vi "dataAcq_get_interferogram_part.vi"(0 "reference":refnum<class "OSA.lvclass">, 5 "error in (no error)":errorcluster) -> (14 "duplicate reference":refnum<class "OSA.lvclass">, 19 "error out":errorcluster)   [LabVIEW 2010, in "OSA.lvclass"]
doc: "Reads data from spectrometer and updates interferogram Y array, X is equidistant and only x min and max are retrieved. \n\nX: optical path length\nY: ADC value\n\nServes mainly compatibility issues - not recommended for new design/vis."
uses:
  OSA.lvclass
  OSA20X_misc.lvlib
  FTSLib.dll
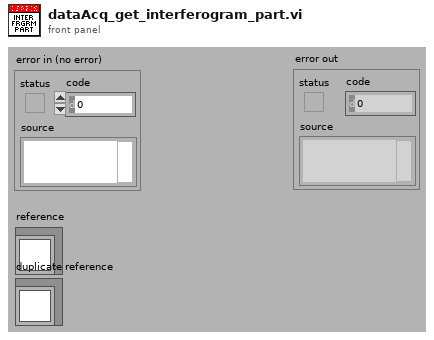
[diagram p1: front panel]
types:
  T1 = enum16{"get", "init", "set interferogram", "set spectrum", "cleanUp"}
  T2 = typedef "OSA.lvclass/ObjectAttributes.ctl" = cluster{"Stop":bool, "dataType":T3, "spectrometerIdx":u16, "buffer size interferogram":i32, "interferogram":cluster{"new":bool, "plot_x_ min":sgl, "plot_x_max":sgl, "plot_y_min":sgl, "plot_y_max":sgl, "Graph Intrfrgrm":T4, "timeStamp":u32, "signal (%)":dbl, "traces":cluster{"idx":u32, "broadBand":bool, "monoChromatic":bool, "peakToPeakSignal":dbl, "peakToPeakPos":dbl}[], "traces idx last":i32}, "spectrum":cluster{"new":bool, "plot_x_min":sgl, "plot_x_max":sgl, "plot_unit_x":T5, "plot_unit_y":T6, "plot_y_min":sgl, "plot_y_max":sgl, "Graph Spectrum":T4, "timeStamp":u32, "X_VAL_OPTIONS":enum16{"MIN_MAX", "ARRAY"}, "traces":cluster{"idx":u32}[], "traces idx last":i32}, "Thorlabs_OSA_64.lvclass:queue_action.ctlqueue ref":refnum<queue>, "action":T7, "plot zoom step":dbl, "buffer semaphore":T8, "acq stopped":bool, "dataType active":T3, "temperature (degr C)":sgl, "pressure (hPa)":sgl, "rel humidity (%)":sgl, "settings":cluster{"resolution":u16, "sensitivity":u16, "Average":bool, "average nr":u32, "apodisation":T9, "acq delay (ms)":u32, "airMesure":T10, "wmtr on":bool, "intfgrm_smooth_width":u16, "intfgrm_smooth_nrOfPasses":u16, "intfgrm_smooth":T11, "phaseCorrection":T12, "zeroFill":u8, "spectr_smooth":T11, "spectr_smooth_width":u16, "spectr_smooth_nrOfPasses":u16, "resolution (/cm)":sgl, "REF wavelength, (nm)":dbl, "gain_idx":u16, "gainAuto":bool, "gain_relative":dbl, "PD sensitivity mode":T13, "PD senseMode implemented":bool, "SensorTemperature implemented":bool, "SensorPressure implemented":bool, "SensorHumidity implemented":bool}, "peaks position":sgl[], "peaks width":sgl[], "peaks height":sgl[], "peaks max nr":u32, "peaks latest nr":i32, "peaks new":bool, "power":dbl, "power new":bool, "path":string, "wavelength (WNr)":dbl, "wavelength new":bool, "buffer size spectrum":i32, "status":string, "VI reference":refnum<vi>, "funcPointer":u64, "libraryPointer":u64, "singleAcquisition":bool, "coherenceLength (cm)":dbl, "coherenceLength new":bool, "spectrometer model":string, "spectrometer serial nr":string, "peaks thld left":sgl[], "peaks thld right":sgl[], "coherenceLength error (cm)":dbl, "ADC bits":u16, "peaks position centroid":sgl[], "peaks height centroid":sgl[], "OSA series":T14, "channel index spectrum":u16, "spectrometer rangeLow, (/cm)":dbl, "spectrometer rangeHigh, (/cm)":dbl, "channel index interferogram":u16}
  T3 = typedef "OSA.lvclass/acq_dataType.ctl" = enum16{"none", "interferogram", "spectrum"}
  T4 = typedef "OSA.lvclass/graph_intensity.ctl" = refnum<vi>
  T5 = typedef "OSA.lvclass/spectrum_x_unit.ctl" = enum16{"wavenr/cm", "THz", "eV", "nm_air", "nm_vac"}
  T6 = typedef "OSA.lvclass/y_unit.ctl" = enum16{"ADC counts", "dBm pwr absolute", "dBm pwr density", "mW pwr absolute", "mW pwr density"}
  T7 = typedef "OSA.lvclass/queue_action.ctl" = enum16{"none", "stop", "GUI_plotInterferogram", "GUI_plotSpectrum", "GUI_plotInterferogramRescale", "GUI_plotSpectrumRescale", "GUI_plotInterferogramReset", "GUI_plotSpectrumReset", "GUI_plotInterferogramAutoScaleY", "GUI_plotSpectrumAutoScaleY", "GUI_plotInterferogramZoomOut", "GUI_plotSpectrumZoomOut", "GUI_plotInterferogramPane", "GUI_plotSpectrumPane", "GUI_plotInterferogramZoomMouse", "GUI_plotSpectrumZoomMouse", "ENVIRONMENT temperature", "ENVIRONMENT pressure", "MODE_resolution set", "MODE_resolution get", "MODE_sensitivity set", "MODE_sensitivity get", "MODE_PDTemperature set", "MODE_PDTemperature get", "REBOOT/RESET firmware", "ACQASYNC_acquireSingleSpectrum", "ACQASYNC_continuous start", "ACQASYNC_continuous stop\n", "ACQASYNC_get last interferogram", "ACQASYNC_get last spectrum", "ACQASYNC_get last waveNr", "ACQOPT_interferogram smoothing set", "ACQOPT_interferogram smoothing get", "ACQOPT_spectrum smoothing set", "ACQOPT_spectrum smoothing get", "ACQOPT_apodisation type set", "ACQOPT_apodisation type get", "ACQOPT_phase correction type set", "ACQOPT_phase correction type get", "ACQOPT_acqIntervall_set", "ACQOPT_acqIntervall_get", "ACQOPT_average spectrum set", "ACQOPT_average spectrum get", "ACQOPT_rolling average set", "ACQOPT_rolling average get", "ACQOPT_zero fill factor set", "ACQOPT_zero fill factor get", "ACQOPT_cycle counting set", "ACQOPT_cycle counting get", "ACQOPT_air measure option set", "ACQOPT_air measure option get", "ACQOPT_gainLevel auto get", "ACQOPT_gainLevel auto set", "ACQOPT_gainLevel get", "ACQOPT_gainLevel set", "ACQOPT_getAll", "INSTRUMENT_PROPERTY_range_WaveNr_min", "INSTRUMENT_PROPERTY_range_WaveNr_max", "INSTRUMENT_PROPERTY_reference_wavelength_cm^-1", "INSTRUMENT_PROPERTY_samplesPerRefPeriod", "INSTRUMENT_PROPERTY_resolution_waveNrPercm", "INSTRUMENT_PROPERTY_availableGainLevels", "INSTRUMENT_PROPERTY_status", "CONVERT", "ANALYSE_POWER", "ANALYSE_PEAKS", "ANALYSE_WAVELENGTH", "ANALYSE_SPECTRUM", "ANALYSE_INTERFEROGRAM", "ANALYSE_COHERENCE_LENGTH", "MATH", "MATH_power", "MATH_peaks", "FILE", "miscellaneous"}
  T8 = typedef "Semaphore RefNum" = refnum<k1>
  T9 = typedef "OSA.lvclass/apodisation.ctl" = enum16{"NONE", "NORTON_BEER_WEAK", "NORTON_BEER_MEDIUM", "NORTON_BEER_STRONG", "TRIANGULAR", "COSINE", "HANN", "HAMMING", "BLACKMANHARRIS3", "BLACKMANHARRIS4", "GAUSSIAN"}
  T10 = typedef "OSA.lvclass/airMeasure.ctl" = enum16{"TEMPERATURE", "PRESSURE"}
  T11 = typedef "OSA20X_misc.lvlib/interferogram_smoothing.ctl" = enum16{"NONE", "BINOMIAL", "SAVITSKY_GOLAY", "FOURIER", "MOVING_AVERAGE", "GAUSSIAN"}
  T12 = typedef "OSA.lvclass/phaseCorrection.ctl" = enum16{"NONE", "MERTZ", "FORMAN", "MERTZ_FILE", "FORMAN_FILE", "FUTURE COMP."}
  T13 = typedef "OSA20X_misc.lvlib/PDTemperatureMode.ctl" = enum16{"cool: better sensitivity/noise floor", "warm: extended wl range"}
  T14 = typedef "OSA.lvclass/OSA_series.ctl" = enum16{"OSA200", "OSA300", "UNKNOWN"}
  T15 = cluster{"length":u32, "X min (cm)":sgl, "X max (cm)":sgl, "saturated":bool, "broadband":bool, "isMonoChromatic":bool, "peakToPeak, (counts)":dbl, "peakToPeak position (cm)":dbl, "samplesPerRefPeriod":i32}
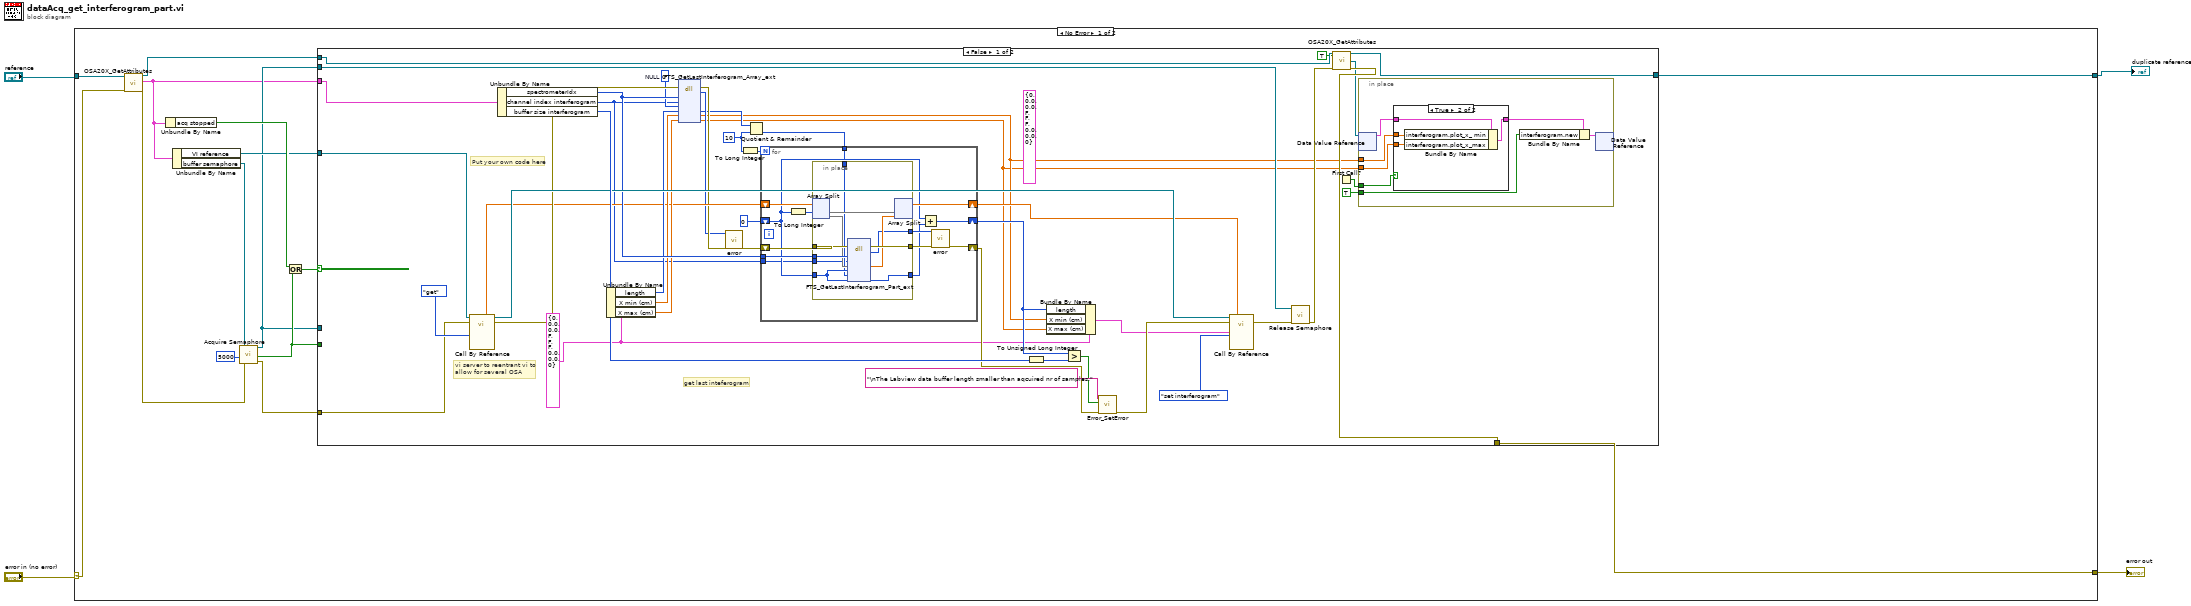
[diagram p0: block diagram]
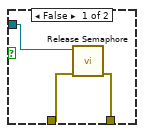
[diagram p4: hidden frame]
diagram:
  n1 = case shown="No Error" "error in (no error)" {
    selector: "error in (no error)" -> [w18 w110]
    tunnel: [w17 w110] -> w3
    tunnel: "reference" -> [w19 w109]
    tunnel: [w16 w109] -> w1
    frame No Error {
      n2 = call "OSA20X_GetAttributes.vi"("reference in"=w19, "error in (no error)"=w18) -> ("reference out"=w8:refnum<class "OSA.lvclass">, "Data"=w5:T2, "error out"=w12:errorcluster)  [unwired: 14 in, 1 out]
      n3 = Unbundle By Name(w5) -> ("acq stopped"=w15:bool)
      n4 = Unbundle By Name(w5) -> ("VI reference"=w9:refnum<vi>, "buffer semaphore"=w13:T8)
      n5 = call <vilib>:"Acquire Semaphore.vi"("error in (no error)"=w12, "ms timeout (-1)"=5000, "semaphore"=w13) -> ("error out"=w10:errorcluster, "timed out"=w7:bool, "semaphore out"=w6:T8)  [unwired: 2 in]
      n6 = Or(x=w15, y=w7) -> (x .or. y?=w14:bool)
      n7 = case shown="False" w14 {
        tunnel: w5 -> [w63 _]
        tunnel: w10 -> [w50 w101]
        tunnel: [w60 w100] -> w17
        tunnel: [w59 w104] -> w16
        tunnel: w6 -> [w52 _]
        tunnel: w9 -> [w49 _]
        tunnel: w8 -> [w47 w104]
        tunnel: w7 -> [_ w103]
        tunnel: w6 -> [_ w102]
        frame False {
          w22 = T15 {"length"=0, "X min (cm)"=0.0, "X max (cm)"=0.0, "saturated"=FALSE, "broadband"=FALSE, "isMonoChromatic"=FALSE, "peakToPeak, (counts)"=0.0, "peakToPeak position (cm)"=0.0, "samplesPerRefPeriod"=0} ("interferogram prop set")
          (unwired) T15 {"length"=0, "X min (cm)"=0.0, "X max (cm)"=0.0, "saturated"=FALSE, "broadband"=FALSE, "isMonoChromatic"=FALSE, "peakToPeak, (counts)"=0.0, "peakToPeak position (cm)"=0.0, "samplesPerRefPeriod"=0} ("interferogram prop set")
          w34 = u32 10 ("y")
          w40 = i64 0  # NULL
          # "get last inteferogram"
          # "vi server to reentrant vi to \nallow for several OSA"
          # "Put your own code here"
          n8 = call-by-ref "?"(reference=w49, error in=w50, "action"=T1."get") -> (reference out=w48:refnum<vi>, error out=w41:errorcluster, "interferogram"=w36:sgl[])  [unwired: 14 in, 4 out]
          n9 = Unbundle By Name(w63) -> ("spectrometerIdx"=w42:u16, "channel index interferogram"=w20:u16, "buffer size interferogram"=w58:i32)
          n10 = Unbundle By Name(w22) -> ("length"=w37:u32, "X min (cm)"=w39:sgl, "X max (cm)"=w38:sgl)
          n11 = dll-call lib="FTSLib.dll" fn="FTS_GetLastInterferogram_Array_ext"(error in=w41, "spectrIdx"=w42, "channel"=w20, "spec"=w40, "length"=w37, "x_min"=w39, "x_max"=w38) -> (error out=w32:errorcluster, "return type"=w30:i32, "length"=w27:u32, "x_min"=w24:sgl, "x_max"=w23:sgl)  [unwired: 5 in, 1 out]
          n12 = call "error.vi"("result code"=w30, "error in (no error)"=w32) -> ("error out"=w31:errorcluster)  [unwired: 15 in, 2 out]
          n13 = To Long Integer(number=w34) -> (32bit integer=w28:i32)
          n14 = Quotient & Remainder(x=w27, y=w34) -> (floor(x/y)=w29:u32)  [unwired: 1 out]
          n15 = for {
            N: w28 -> [_]
            tunnel: w42 -> [w73]
            shift-right: [w75] -> w35
            shift-left: w36 -> [w76]
            shift-right: [w71] -> w25
            shift-left: w31 -> [w74]
            shift-right: [w66] -> w26
            shift-left: u32 0 ("y") -> [w67]
            tunnel: w29 -> [w65]
            tunnel: w20 -> [w64]
            n16 = To Long Integer(number=w67) -> (32bit integer=w70:i32)
            n17 = in-place {
              in-place-border: w73 -> [w87]
              in-place-border: w74 -> [w86]
              in-place-border: [w85] -> w72
              in-place-border: [w81] -> w69
              in-place-border: [w80] -> w68
              in-place-border: w67 -> [w79]
              in-place-border: w65 -> [w78]
              in-place-border: w64 -> [w77]
              n18 = in-place-split #1(w76, w70) -> (w84:sgl[], w83:sgl[])
              n19 = dll-call lib="FTSLib.dll" fn="FTS_GetLastInterferogram_Part_ext"(error in=w86, "spectrIdx"=w87, "channel"=w77, "spec"=w83, "idxStart"=w79, "length"=w78, "valuesUpdated"=w79) -> (error out=w85:errorcluster, "return type"=w81:i32, "spec"=w82:sgl[], "valuesUpdated"=w80:u32)  [unwired: 6 in, 1 out]
              n20 = in-place-split #1(w84, w82) -> (w75:sgl[])  [unwired: 1 out]
            }
            n21 = Add(x=w67, y=w68) -> (x+y=w66:u32)
            n22 = call "error.vi"("result code"=w69, "error in (no error)"=w72) -> ("error out"=w71:errorcluster)  [unwired: 15 in, 2 out]
          }
          n23 = To Unsigned Long Integer(number=w58) -> (unsigned 32bit integer=w57:u32)
          n24 = Bundle By Name(cluster=w22, "length"=w26, "X min (cm)"=w24, "X max (cm)"=w23) -> (w21:T15)
          n25 = Greater?(x=w26, y=w57) -> (0:w61:bool)
          n26 = call "Error_SetError.vi"("error in"=w25, "status (true)"=w61, "source(\"\")"="\nThe Labview data buffer length smaller than aqcuired nr of samples." ("source(\"\")")) -> ("error out"=w54:errorcluster)  [unwired: 4 in]
          n27 = call-by-ref "?"(reference=w48, error in=w54, "interferogram prop set"=w21, "action"=T1."set interferogram", "interferogram set"=w35) -> (error out=w53:errorcluster)  [unwired: 12 in, 6 out]
          n28 = call <vilib>:"Release Semaphore.vi"("error in (no error)"=w53, "semaphore"=w52) -> ("error out"=w55:errorcluster)  [unwired: 4 in, 1 out]
          n29 = call "OSA20X_GetAttributes.vi"("reference in"=w47, "OnlyGetDvrReference(False)"=TRUE, "error in (no error)"=w55) -> ("reference out"=w59:refnum<class "OSA.lvclass">, "DataRef"=w45:refnum<data-value>, "error out"=w60:errorcluster)  [unwired: 13 in, 1 out]
          n30 = First Call?() -> (First Call?: T/F=w44:bool)
          n31 = in-place {
            in-place-border: w44 -> [w94]
            in-place-border: w24 -> [w92]
            in-place-border: w23 -> [w91]
            in-place-border: TRUE ("interferogram.new") -> [w89]
            n32 = in-place-dvr #2(w45) -> (w93:T2)  [unwired: 1 out]
            n33 = case shown="True" w94 {
              tunnel: w93 -> [w95 w99]
              tunnel: [w95 w98] -> w90
              tunnel: w92 -> [_ w97]
              tunnel: w91 -> [_ w96]
              frame False {
              }
              frame True {
                n34 = Bundle By Name(cluster=w99, "interferogram.plot_x_ min"=w97, "interferogram.plot_x_max"=w96) -> (w98:T2)
              }
            }
            n35 = Bundle By Name(cluster=w90, "interferogram.new"=w89) -> (w88:T2)
            n36 = in-place-dvr #2(w88) -> ()  [unwired: 2 out]
          }
        }
        frame True {
          n37 = case shown="True" w103 {
            tunnel: w102 -> [w107 _]
            tunnel: w101 -> [w106 w108]
            tunnel: [w105 w108] -> w100
            frame False {
              n38 = call <vilib>:"Release Semaphore.vi"("error in (no error)"=w106, "semaphore"=w107) -> ("error out"=w105:errorcluster)  [unwired: 4 in, 1 out]
            }
            frame True {
            }
          }
        }
      }
    }
    frame Error {
      # "Error"
    }
  }
  "error out" <- w3
  "duplicate reference" <- w1
